vi "PT1.vi"(10 "Zeitkonstante(Tau)":dbl, 11 "Eingang":dbl) -> (3 "Ausgang":dbl)   [LabVIEW 2015]
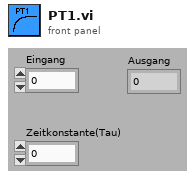
[diagram p1: front panel]
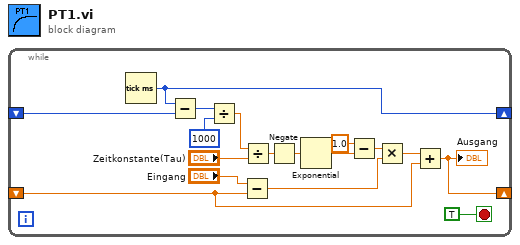
[diagram p0: block diagram]
diagram:
  n1 = while {
    shift-right: [w16] -> _
    shift-left: _ -> [w17]
    shift-right: [w3] -> _
    shift-left: _ -> [w1]
    stop <- TRUE stop-if-true
    n2 = Tick Count (ms)() -> (millisecond timer value=w16:u32)
    n3 = Subtract(x=w16, y=w17) -> (x-y=w14:u32)
    n4 = Divide(x=w14, y=u32 1000) -> (x/y=w10:dbl)
    n5 = Subtract(x="Eingang", y=w1) -> (x-y=w5:dbl)
    n6 = Divide(x=w10, y="Zeitkonstante(Tau)") -> (x/y=w7:dbl)
    n7 = Negate(x=w7) -> (-x=w6:dbl)
    n8 = Exponential(1:w6) -> (0:w11:dbl)
    n9 = Subtract(x=1.0, y=w11) -> (x-y=w8:dbl)
    n10 = Multiply(x=w8, y=w5) -> (x*y=w2:dbl)
    n11 = Add(x=w2, y=w1) -> (x+y=w3:dbl)
    "Ausgang" <- w3
  }
